vi "Diagnose Zykluszeit.vi"() -> ()   [LabVIEW 2020, in "allgemeine Sub-VIs.lvlib"]
uses:
  allgemeine Sub-VIs.lvlib
  Zykluszeiterfassung Aktionen.ctl
  Seiten/FT-IR/Get Spectra/Aktion FGV Background-Daten.ctl
  Seiten/FT-IR/Get Spectra/Get Spectra.lvlib
  Seiten/FT-IR/AK interface/AK-Interface.lvlib
panel:
  out "AK Extern Hz":sgl=80.0 caption="Hz" format="%#.1f"
  out "AK - FT-IR Hz":sgl=80.0 caption="Hz" format="%#.1f"
  out "ToolWeb Hz":sgl=80.0 caption="Hz" format="%#.1f"
  out "AK - Extern":sgl=80.0 format="%#.1f"
  out "AK - FT-IR":sgl=80.0 format="%#.1f"
  out "ToolWeb":sgl=80.0 format="%#.1f"
  out "Messdaten":sgl=80.0 format="%#.1f"
  out "Messdaten Hz":sgl=80.0 caption="Hz" format="%#.1f"
  in  "Stopp":bool
  # "Diagnose Zykluszeit"
  # "ms"
  # "ms"
  # "ms"
  # "ms"
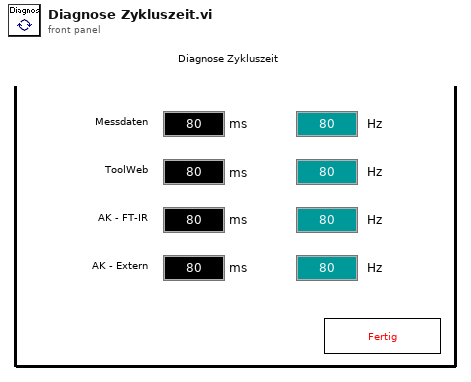
[diagram p1: front panel]
types:
  T1 = typedef "allgemeine Sub-VIs.lvlib/Zykluszeiterfassung Aktionen.ctl" = enum16{"lesen", "init", "Messdaten1", "ToolWeb", "AK FT-IR", "AK Extern", "AK Amium"}
  T2 = typedef "FT-IR.lvlib/Get Spectra.lvlib/Aktion FGV Background-Daten.ctl" = enum16{"lesen", "schreiben", "Background aktiv", "Referenz", "laden", "speichern", "Plot sichtbar"}
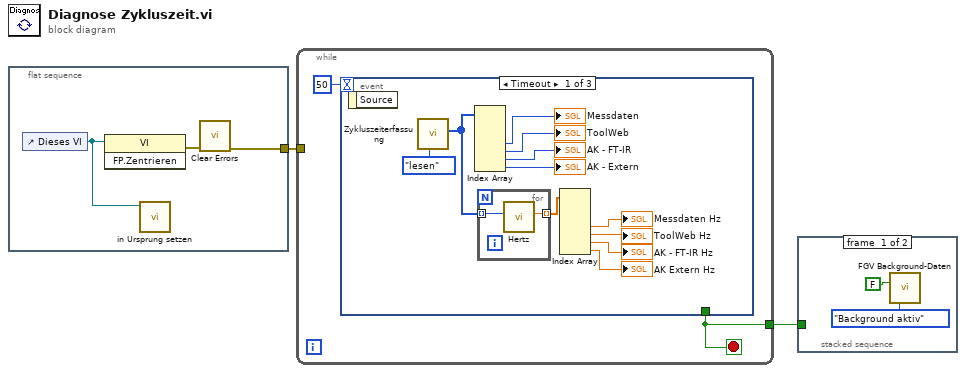
[diagram p0: block diagram]
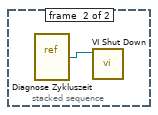
[diagram p2: hidden frame]
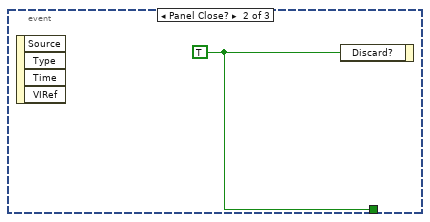
[diagram p3: hidden frame]
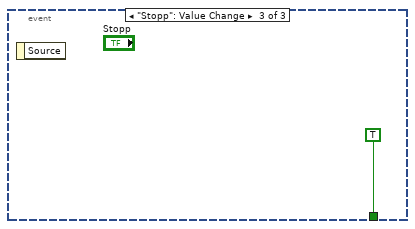
[diagram p4: hidden frame]
diagram:
  n1 = flat-sequence {
    tunnel: [w4] -> w1
    frame #0 {
      n2 = control-ref of="Dieses VI"() -> (w3:refnum<vi>)
      n3 = invoke class="VI" method="FP.Zentrieren"(reference=w3) -> (error out=w5:errorcluster)  [unwired: 2 in, 2 out]
      n4 = call "in Ursprung setzen.vi"("VI Referenz"=w3) -> ()  [unwired: 10 in, 1 out]
      n5 = call <vilib>:"Clear Errors.vi"("error in (no error)"=w5) -> ("error out"=w4:errorcluster)  [unwired: 5 in, 1 out]
    }
  }
  n6 = while {
    tunnel: [w6] -> w2
    tunnel: w1 -> [_]
    stop <- w6 stop-if-true
    n7 = event shown="[0] Timeout" {
      selector: _ -> [_ _ _]
      dyn-events: _ -> [_ _ _]
      timeout: 50 -> [_ _ _]
      tunnel: [_ w21 TRUE ("Verwerfen?")] -> w6
      event Timeout {
        n8 = event-data() -> ()  [unwired: 1 in, 1 out]
        n9 = call "Zykluszeiterfassung.vi"("Aktionen"=Zykluszeiterfassung_Aktionen."lesen") -> ("Zykluszeiten"=w17:u32[])  [unwired: 10 in]
        n10 = Index Array(array=w17) -> (element #3=→"Messdaten":u32, element #4=→"ToolWeb":u32, element #5=→"AK - FT-IR":u32, element #6=→"AK - Extern":u32)  [unwired: 6 in, 2 out]
        n11 = for {
          tunnel: w17 -> [w20] mode=indexing
          tunnel: [w19] -> w16 mode=indexing
          n12 = call "Hertz.vi"("Zeit [ms]"=w20) -> ("Hertz"=w19:sgl)  [unwired: 10 in]
        }
        n13 = Index Array(array=w16) -> (element #3=→"Messdaten Hz":sgl, element #4=→"ToolWeb Hz":sgl, element #5=→"AK - FT-IR Hz":sgl, element #6=→"AK Extern Hz":sgl)  [unwired: 6 in, 2 out]
      }
      event Panel Close? {
        w21 = TRUE ("Verwerfen?")
        n14 = event-data() -> ()  [unwired: 1 in, 4 out]
        n15 = event-data("Discard?"=w21) -> ()  [unwired: 1 in, 1 out]
      }
      event "Stopp": Value Change {
        n16 = event-data() -> ()  [unwired: 1 in, 1 out]
      }
    }
  }
  n17 = stacked-sequence {
    tunnel: w2 -> [_ _]
    frame #0 {
      n18 = call "FGV Background-Daten.vi"("Background aktiv"=FALSE, "Aktion"=Aktion_FGV_Background-Daten."Background aktiv") -> ()  [unwired: 6 in, 8 out]
    }
    frame #1 {
      n19 = vi-ref "Diagnose Zykluszeit.vi"() -> (w25:refnum<vi>)
      n20 = call "VI Shut Down.vi"("VI Referenz"=w25) -> ()  [unwired: 11 in]
    }
  }
